vi "test_CHROMA.vi"   [LabVIEW 2012]
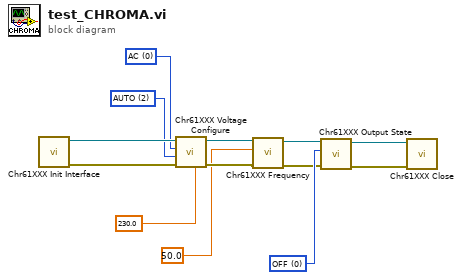
[diagram p0: block diagram]
diagram:
  w9 = 2 items=["LOW", "HIGH", "AUTO"] ("voltage range")
  w8 = 0 items=["AC", "DC"] ("voltage type")
  w5 = u16 0 items=["OFF", "ON"] ("state")
  n1 = call <vilib>:"Chr61XXX Init Interface.vi"() -> ("error out"=w10:errorcluster, "instrument handle out"=w11:refnum<k15>)  [unwired: 9 in, 1 out]
  n2 = call <vilib>:"Chr61XXX Voltage Configure.vi"("voltage"=230.0, "error in (no error)"=w10, "voltage range"=w9, "voltage type"=w8, "instrument handle"=w11) -> ("error out"=w4:errorcluster, "instrument handle out"=w7:refnum<k15>)  [unwired: 5 in]
  n3 = call <vilib>:"Chr61XXX Frequency.vi"("error in (no error)"=w4, "frequency"=50.0 ("voltage"), "instrument handle"=w7) -> ("error out"=w3:errorcluster, "instrument handle out"=w6:refnum<k15>)  [unwired: 7 in]
  n4 = call <vilib>:"Chr61XXX Output State.vi"("error in (no error)"=w3, "state"=w5, "instrument handle"=w6) -> ("error out"=w12:errorcluster, "instrument handle out"=w13:refnum<k15>)  [unwired: 7 in]
  n5 = call <vilib>:"Chr61XXX Close.vi"("error in (no error)"=w12, "instrument handle"=w13) -> ()  [unwired: 9 in, 1 out]
